vi "ReadMediaPlayer.vi"(0 "reference in":refnum<class "MusicPlayer.lvclass">, 11 "Error In":errorcluster) -> (4 "reference out":refnum<class "MusicPlayer.lvclass">, 8 "MediaPlayer":refnum<k7>, 15 "Error Out":errorcluster)   [LabVIEW 2022 SP3, in "MusicPlayer.lvclass"]
uses:
  MusicPlayer.lvclass
  MusicPlayer.lvclass/MusicPlayer.ctl
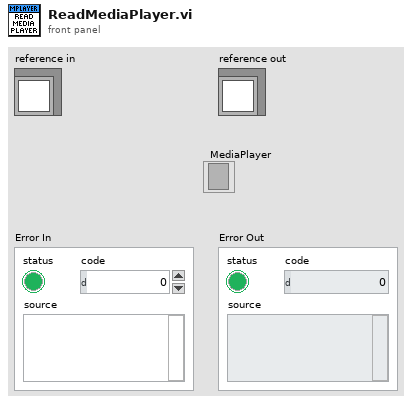
[diagram p1: front panel]
types:
  T1 = typedef "MusicPlayer.lvclass/ObjectAttributes.ctl" = cluster{"MediaPlayer":refnum<k7>}
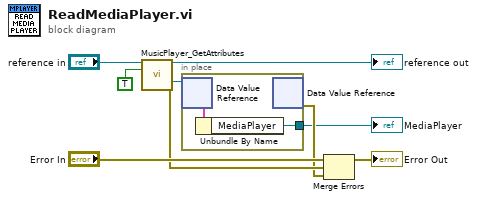
[diagram p0: block diagram]
diagram:
  n1 = call "MusicPlayer_GetAttributes.vi"("reference in"="reference in", "OnlyGetDvrReference(False)"=TRUE) -> ("reference out"=→"reference out":refnum<class "MusicPlayer.lvclass">, "DataRef"=w2:refnum<data-value>, "error out"=w8:errorcluster)  [unwired: 10 in, 1 out]
  n2 = in-place {
    in-place-border: [w11] -> w1
    n3 = in-place-dvr #1(w2) -> (w10:T1)  [unwired: 1 out]
    n4 = Unbundle By Name(w10) -> ("MediaPlayer"=w11:refnum<k7>)
    n5 = in-place-dvr #1() -> (w6:errorcluster)  [unwired: 1 in, 1 out]
  }
  "MediaPlayer" <- w1
  n6 = Merge Errors("Error In", w8, w6) -> (→"Error Out":errorcluster)
